vi "midiOutPlayer.msg.Stop.vi"(8 "error in (no error)":errorcluster, 11 "midi in":refnum<class "midi.lvclass">) -> (0 "error out":errorcluster, 3 "midi out":refnum<class "midi.lvclass">)   [LabVIEW 2020, in "midi.lvclass"]
uses:
  midi.lvclass
  midi.lvclass/midi.ctl
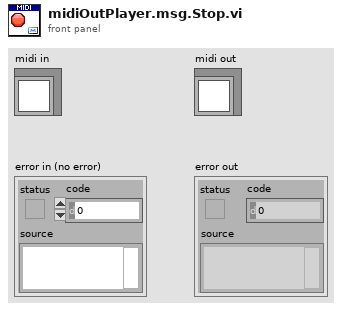
[diagram p1: front panel]
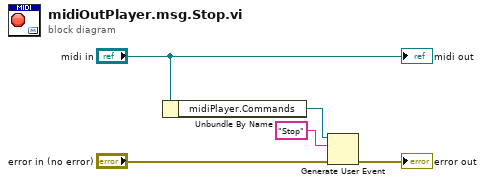
[diagram p0: block diagram]
diagram:
  n1 = Unbundle By Name("midi in") -> ("midiPlayer.Commands"=w5:refnum<user-event>)
  n2 = Generate User Event(user event=w5, event data cluster="Stop" ("event data"), error in="error in (no error)") -> (error out=→"error out":errorcluster)  [unwired: 1 in, 1 out]
  "midi out" <- "midi in"
